vi "Zaber Intermediate - Read Response Data.vi"() -> ()   [LabVIEW 2015]
doc: "Most commands return some kind of data, and you can use that data. In this example, we check that there is room for the movement before starting. This example introduces the Unbundle By Name function.\nNote that not all commands are included in the drop down list. This example uses command 53: Return Setting with command 45: Set Current Position as the data value. To use a command that's not in the drop down list, select <Other>... and then type the command number. See your user manual for a complete list of Zaber motion device commands or joystick commands."
uses:
  ZaberTSeries.lvlib
  Public/Utility/Response.ctl
panel:
  out "Responses":T1[](array[typedef]) {"Command" items=["Constant Speed Tracking"=8, "Echo"=55, "Error"=255, "Home"=1, "Limit Active"=9, "Manual Move Tracking"=10, "Move Absolute"=20, "Move at Constant Speed"=22, "Move Relative"=21, "Renumber"=2, "Restore Settings"=36, "Stop"=23]}
  in  "Move Size":u32=10000
  in  "Device Number":u8=1
  in  "Move count":i32=5
  in  "VISA resource name":refnum<visa-resource-name>
  # "This does the same thing as the previous example, but checks to make sure that\nthere is room for the movement before starting.\nType Ctrl-E to see the block diagram."
  # "Don't use device 0."
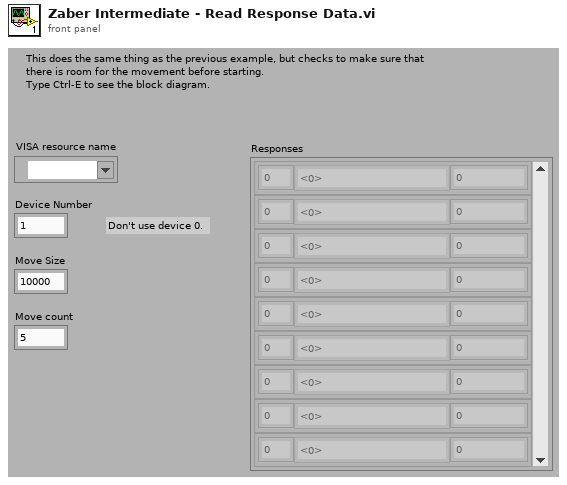
[diagram p1: front panel]
types:
  T1 = typedef "ZaberTSeries.lvlib/Response.ctl" = cluster{"Device Number":u8, "Command":u8, "Data":i32}
  T2 = cluster{"Device Number":u8, "Command":u8, "Data":i32, "Response Count":i32}
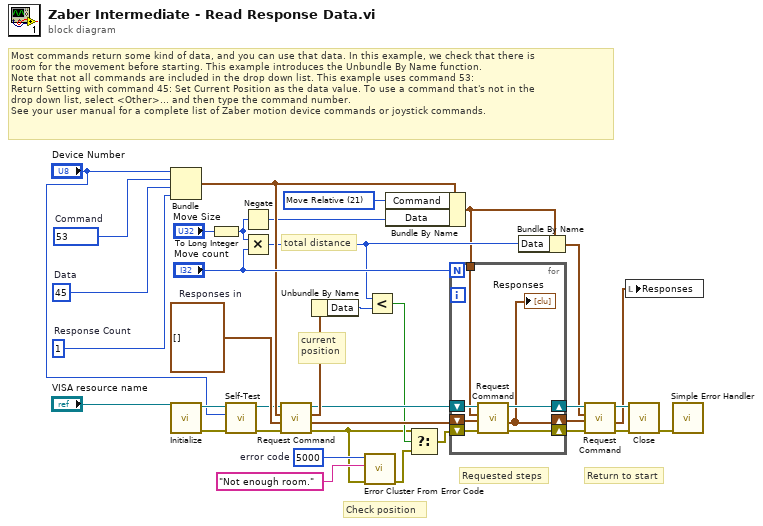
[diagram p0: block diagram]
diagram:
  w10 = 5000  # error code
  w15 = u8 21 items=["Echo"=55, "Home"=1, "Move Absolute"=20, "Move Relative"=21, "Move at Constant Speed"=22, "Renumber"=2, "Restore Settings"=36, "Stop"=23] ("Command")
  w24 = 45  # Data
  w26 = 1  # Response Count
  w27 = u8 53 items=["Echo"=55, "Home"=1, "Move Absolute"=20, "Move Relative"=21, "Move at Constant Speed"=22, "Renumber"=2, "Restore Settings"=36, "Stop"=23]  # Command
  w23 = T1[] []  # Responses in
  # "current\nposition"
  # "total distance"
  # "Most commands return some kind of data, and you can use that data. In this example, we check that there is\nroom for the movement before starting. This example introduces the Unbundle By Name function.\nNote that not all commands are included in the drop down list. This example uses command 53: \nReturn Setting with command 45: Set Current Position as the data value. To use a command that's not in the\ndrop down list, select <Other>... and then type the command number. \nSee your user manual for a complete list of Zaber motion device commands or joystick commands."
  # "Return to start"
  # "Requested steps"
  # "Check position"
  n1 = Bundle("Device Number"="Device Number", "Command"=w27, "Data"=w24, "Response Count"=w26) -> (w19:T2)  [unwired: 1 in]
  n2 = call "Initialize.vi"("VISA resource name"="VISA resource name") -> ("error out"=w5:errorcluster, "VISA resource name out"=w4:refnum<visa-resource-name>)  [unwired: 8 in, 1 out]
  n3 = To Long Integer(number="Move Size") -> (32bit integer=w17:i32)
  n4 = call "Self-Test.vi"("error in (no error)"=w5, "Device Number"="Device Number", "VISA resource name"=w4) -> ("error out"=w3:errorcluster, "VISA resource name out"=w2:refnum<visa-resource-name>)  [unwired: 5 in, 2 out]
  n5 = Negate(x=w17) -> (-x=w18:i32)
  n6 = Multiply(x=w17, y="Move count") -> (x*y=w16:i32)
  n7 = call "Request Command.vi"("error in (no error)"=w3, "Responses in"=w23, "Request"=w19, "VISA resource name"=w2) -> ("error out"=w7:errorcluster, "Responses out"=w12:T1[], "First Response"=w22:T1, "VISA resource name out"=w11:refnum<visa-resource-name>)  [unwired: 4 in]
  n8 = Unbundle By Name(w22) -> ("Data"=w20:i32)
  n9 = call <vilib>:"Error Cluster From Error Code.vi"("error in (no error)"=w7, "error message (\"\")"="Not enough room." ("error message (\"\")"), "error code (0)"=w10) -> ("error out"=w6:errorcluster)  [unwired: 6 in]
  n10 = Less?(x=w16, y=w20) -> (x < y?=w9:bool)
  n11 = Bundle By Name(cluster=w19, "Command"=w15, "Data"=w18) -> (w14:T2)
  n12 = Select(t=w7, s=w9, f=w6) -> (s? t:f=w8:errorcluster)
  n13 = for {
    N: "Move count" -> [_]
    shift-right: [w38] -> w28
    shift-left: w12 -> [w39]
    shift-right: [w40] -> w31
    shift-left: w8 -> [w43]
    tunnel: w14 -> [w37]
    shift-right: [w41] -> w32
    shift-left: w11 -> [w42]
    n14 = call "Request Command.vi"("error in (no error)"=w43, "Responses in"=w39, "Request"=w37, "VISA resource name"=w42) -> ("error out"=w40:errorcluster, "Responses out"=w38:T1[], "VISA resource name out"=w41:refnum<visa-resource-name>)  [unwired: 4 in, 1 out]
    "Responses" <- w38
  }
  n15 = Bundle By Name(cluster=w14, "Data"=w16) -> (w30:T2)
  n16 = call "Request Command.vi"("error in (no error)"=w31, "Responses in"=w28, "Request"=w30, "VISA resource name"=w32) -> ("error out"=w34:errorcluster, "Responses out"=w29:T1[], "VISA resource name out"=w35:refnum<visa-resource-name>)  [unwired: 4 in, 1 out]
  n17 = local write "Responses"(w29) -> ()
  n18 = call "Close.vi"("error in (no error)"=w34, "VISA resource name"=w35) -> ("error out"=w36:errorcluster)  [unwired: 8 in, 1 out]
  n19 = call <vilib>:"Simple Error Handler.vi"("error in (no error)"=w36) -> ()  [unwired: 4 in, 5 out]
